vi "Tuner Analyzer.vi"() -> ()   [LabVIEW 2015]
panel:
  in  "Tab Control":enum32{"Tuner", "Analysis", "Fourier"}(tab)
  out "Note":string
  out "Frequency":dbl
  out "Meter":dbl(knob) scale=-20.0..20.0
  in  "Instrument":string(combo)
  out "XY Graph":cluster{"X":dbl, "Y":dbl}[](graph)
  out "Intensity Graph":dbl[][](graph)
  # "Tuner, note estimation"
  # "Timbre analysis, what instrument"
  # "Fourier Analysis, relative peak intensities, graphs n shit"
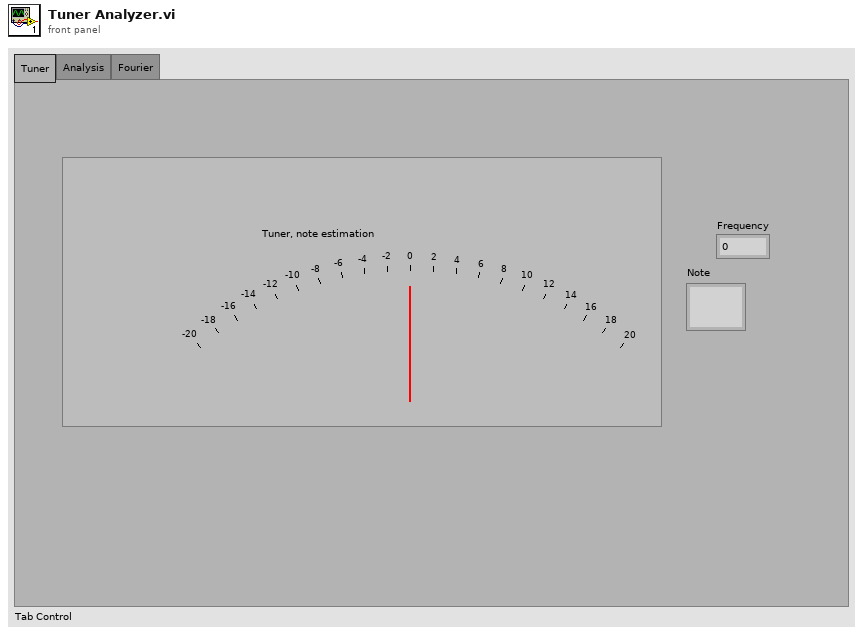
[diagram p1: front panel]
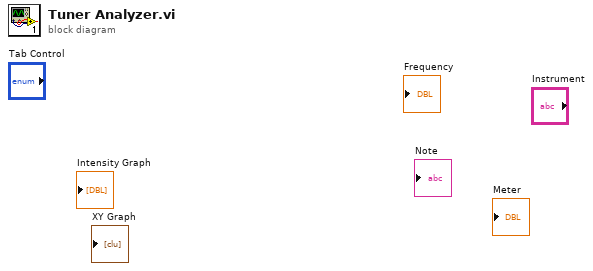
[diagram p0: block diagram]
diagram:
